vi "tlc_Cue Module.vi"(5 "Number of Channels":cluster{"Rows":i32, "Columns":i32}, 6 "Command":T3, 7 "error in (no error)":errorcluster, 8 "Cue Input":T1 {"Channels"."Intensity" min=0.0 max=100.0 step=1.0 format="%#.0f"}, 9 "Swap Index":i32 min=0, 10 "Cue Index":i32 min=0) -> (0 "error out":errorcluster, 1 "Cue Output":T1 {"Channels"."Intensity" min=0.0 max=100.0 step=1.0 format="%#.0f"}, 2 "Number of Cues":i32)   [LabVIEW 2018]
doc: "Controls access to the Cue data."
uses:
  tlc_Cue_Information Command.ctl
  Controls/tlc_Cue_Information.ctl
  Controls/channel.ctl
panel:
  # "Output"
  # "Input"
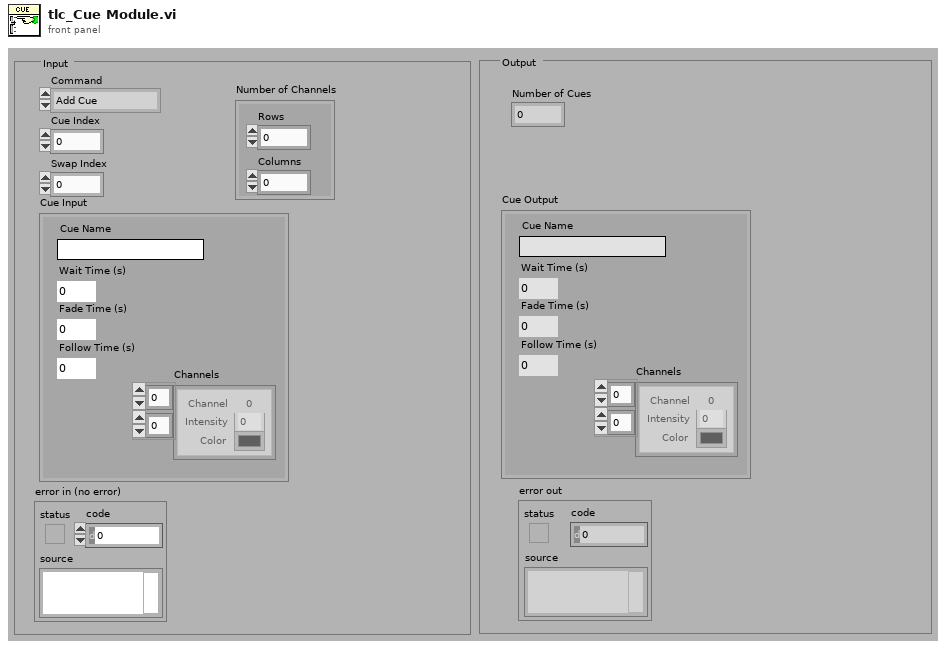
[diagram p1: front panel]
types:
  T1 = typedef "tlc_Cue_Information.ctl" = cluster{"Cue Name":string, "Wait Time (s)":u32, "Fade Time (s)":u32, "Follow Time (s)":u32, "Channels":T2[][]}
  T2 = typedef "channel.ctl" = cluster{"Intensity":dbl, " Color":u32, "Channel":i32}
  T3 = typedef "tlc_Cue_Information Command.ctl" = enum16{"Add Cue", "Delete Cue", "Get Cue Values", "Set Cue Values", "Swap", "Get Number of Cues", "Initialize", "Get Empty Cue"}
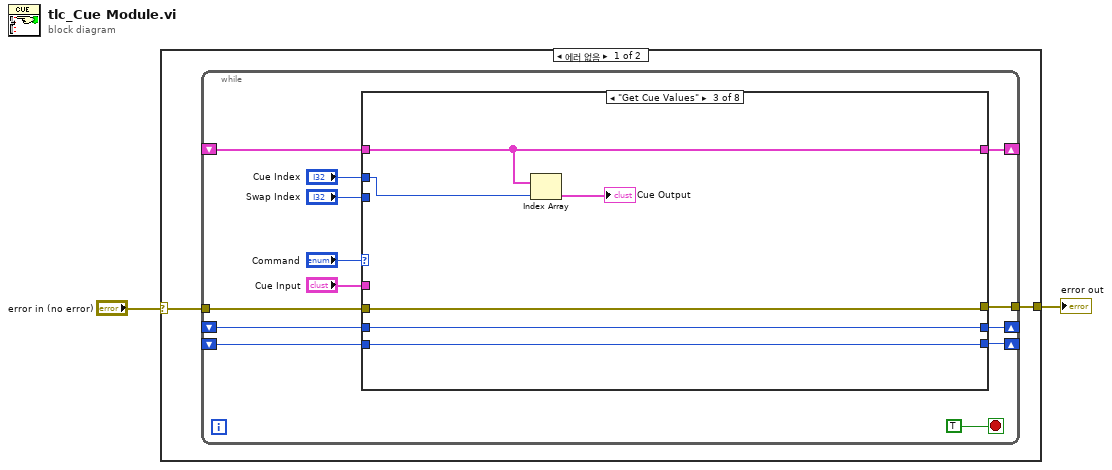
[diagram p0: block diagram]
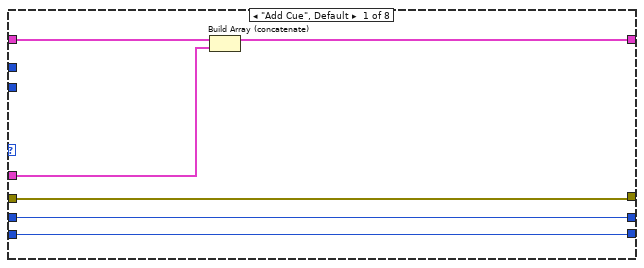
[diagram p2: hidden frame]
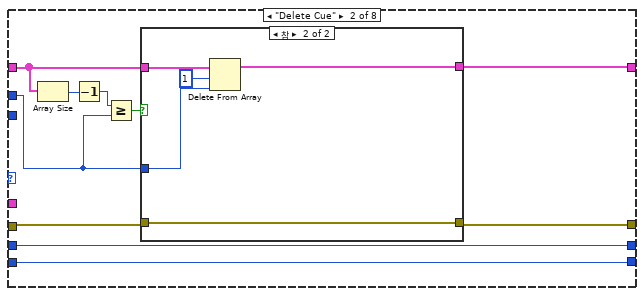
[diagram p3: hidden frame]
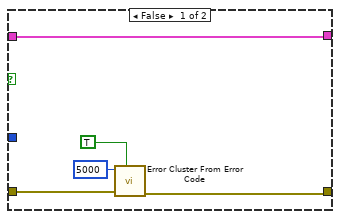
[diagram p4: hidden frame]
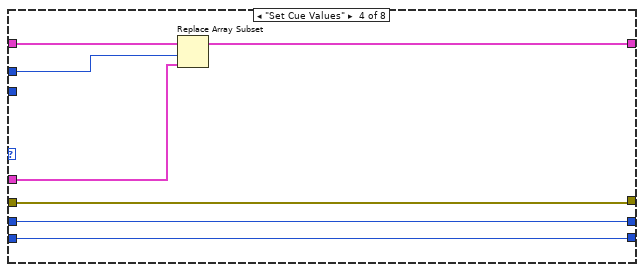
[diagram p5: hidden frame]
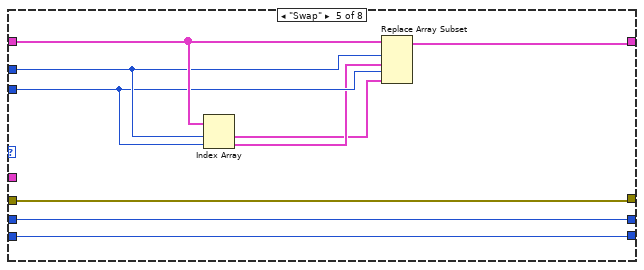
[diagram p6: hidden frame]
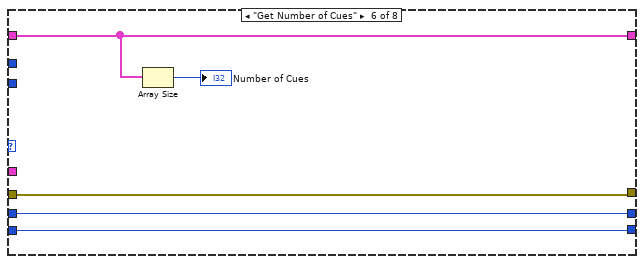
[diagram p7: hidden frame]
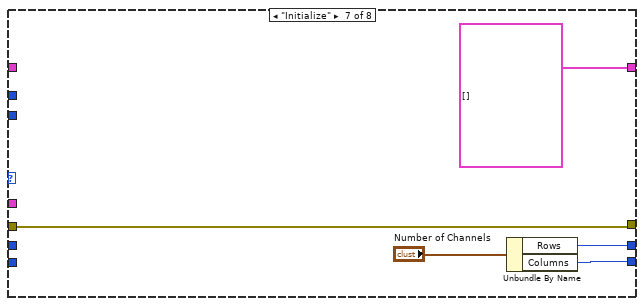
[diagram p8: hidden frame]
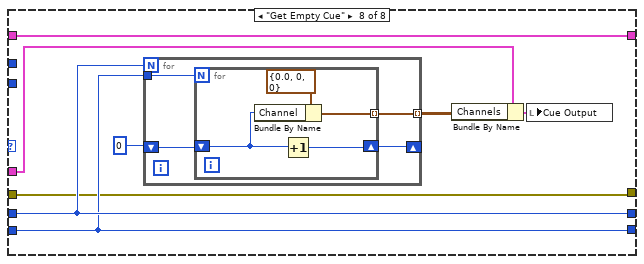
[diagram p9: hidden frame]
diagram:
  n1 = case shown="에러 없음" "error in (no error)" {
    selector: "error in (no error)" -> [w4 w92]
    tunnel: [w3 w92] -> w1
    frame No Error {
      n2 = while {
        shift-right: [w14] -> _
        shift-left: _ -> [w13]
        shift-right: [w10] -> _
        shift-left: _ -> [w8]
        shift-right: [w9] -> _
        shift-left: _ -> [w7]
        tunnel: w4 -> [w6]
        tunnel: [w5] -> w3
        stop <- TRUE stop-if-true
        n3 = case shown="\"Get Cue Values\"" "Command" {
          tunnel: "Cue Input" -> [w23 _ _ w54 _ _ _ w79]
          tunnel: [w22 w33 w49 w55 w60 w70 T1[] [] w80] -> w14
          tunnel: w13 -> [w21 w30 w49 w56 w65 w70 _ w80]
          tunnel: "Cue Index" -> [_ w26 w48 w53 w64 _ _ _]
          tunnel: "Swap Index" -> [_ _ _ _ w63 _ _ _]
          tunnel: [w20 w32 w46 w52 w59 w68 w73 w83] -> w10
          tunnel: [w19 w31 w45 w51 w58 w67 w72 w82] -> w9
          tunnel: w8 -> [w20 w32 w46 w52 w59 w68 _ w83]
          tunnel: w7 -> [w19 w31 w45 w51 w58 w67 _ w82]
          tunnel: w6 -> [w18 w25 w44 w50 w57 w66 w71 w76]
          tunnel: [w18 w24 w44 w50 w57 w66 w71 w76] -> w5
          frame "Add Cue", Default {
            n4 = Build Array (concatenate) "Build Array"(w21, w23) -> (w22:T1[])
          }
          frame "Delete Cue" {
            n5 = Array Size(array=w30) -> (size(s)=w29:i32)
            n6 = Decrement(x=w29) -> (x-1=w27:i32)
            n7 = Greater Or Equal?(x=w27, y=w26) -> (x >= y?=w28:bool)
            n8 = case shown="참" w28 {
              tunnel: w30 -> [w38 w43]
              tunnel: [w38 w42] -> w33
              tunnel: w26 -> [_ w41]
              tunnel: w25 -> [w37 w39]
              tunnel: [w36 w39] -> w24
              frame False {
                n9 = call <vilib>:"Error Cluster From Error Code.vi"("show call chain? (False)"=TRUE, "error in (no error)"=w37, "error code (0)"=5000) -> ("error out"=w36:errorcluster)  [unwired: 6 in]
              }
              frame True {
                n10 = Delete From Array "Delete From Array"(array=w43, length=1, index=w41) -> (array with subset deleted=w42:T1[])  [unwired: 1 out]
              }
            }
          }
          frame "Get Cue Values" {
            n11 = Index Array "Index Array"(array=w49, index=w48) -> (element=→"Cue Output":T1)
          }
          frame "Set Cue Values" {
            n12 = Replace Array Subset "Replace Array Subset"(array=w56, new element=w54, index=w53) -> (w55:T1[])
          }
          frame "Swap" {
            n13 = Index Array "Index Array"(array=w65, index #1=w64, index #2=w63) -> (element #1=w61:T1, element #2=w62:T1)
            n14 = Replace Array Subset "Replace Array Subset"(array=w65, new element #1=w62, index #1=w64, new element #2=w61, index #2=w63) -> (w60:T1[])
          }
          frame "Get Number of Cues" {
            n15 = Array Size(array=w70) -> (size(s)=→"Number of Cues":i32)
          }
          frame "Initialize" {
            n16 = Unbundle By Name("Number of Channels") -> ("Rows"=w73:i32, "Columns"=w72:i32)
          }
          frame "Get Empty Cue" {
            n17 = for {
              N: w83 -> [_]
              tunnel: w82 -> [w87]
              shift-right: [w84] -> _
              shift-left: 0 -> [w86]
              tunnel: [w85] -> w78 mode=indexing
              n18 = for {
                N: w87 -> [_]
                shift-right: [w90] -> w84
                shift-left: w86 -> [w89]
                tunnel: [w88] -> w85 mode=indexing
                n19 = Bundle By Name "Bundle By Name"(cluster=T2 {"Intensity"=0.0, " Color"=0, "Channel"=0} ("UI Channel"), "Channel"=w89) -> (w88:T2)
                n20 = Increment(x=w89) -> (x+1=w90:i32)
              }
            }
            n21 = Bundle By Name "Bundle By Name"(cluster=w79, "Channels"=w78) -> (w77:T1)
            n22 = local write "Cue Output"(w77) -> ()
          }
        }
      }
    }
    frame Error {
    }
  }
  "error out" <- w1
